vi "update file name.vi"(8 "error in":errorcluster, 11 "Picture File in":refnum<class "Picture File.lvclass">) -> (0 "error out":errorcluster, 3 "Picture File out":refnum<class "Picture File.lvclass">)   [LabVIEW 2023, in "File Classes.lvlib" / "Picture File.lvclass"]
uses:
  Picture File.lvclass
  D:/Library/LabVIEW Projects/Personal projects/Picture Organiser/PictureOrganizer/File Classes/File/File.lvclass
  Picture File.lvclass/Picture File.ctl
  File/File.lvclass/File.ctl
  File/Accessors/Read destination path.vi
  File/Accessors/Read file format.vi
  File/Read event name.vi
  File/Accessors/Read file extension.vi
  File/Accessors/Write new destination.vi
  File/File.lvclass
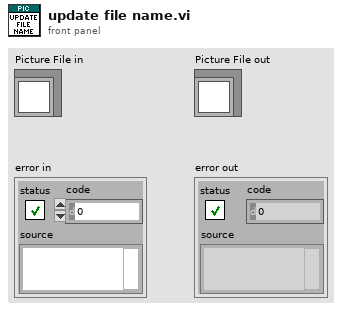
[diagram p1: front panel]
types:
  T1 = typedef "File Classes.lvlib/exif data cluster.ctl" = cluster{"Make":string, "Model":string, "Orientation":u16, "Date":timestamp, "Width":u16, "Height":u16, "Square?":bool, "File Name":string, "Extension":string, "Valid?":bool, "Path":path, "size":i64, "No Ext?":bool, "prefix?":bool, "Tag":string, "Name Type":T2, "Projection Type":string}
  T2 = typedef "File Classes.lvlib/rename type enum.ctl" = enum16{"Date & Time (Default)", "Model Sufix", "Event Sufix", "Model & Event Sufix"}
  T3 = enum16{"Date & Time (Default)", "Model Sufix", "Event Sufix", "Model & Event Sufix"}
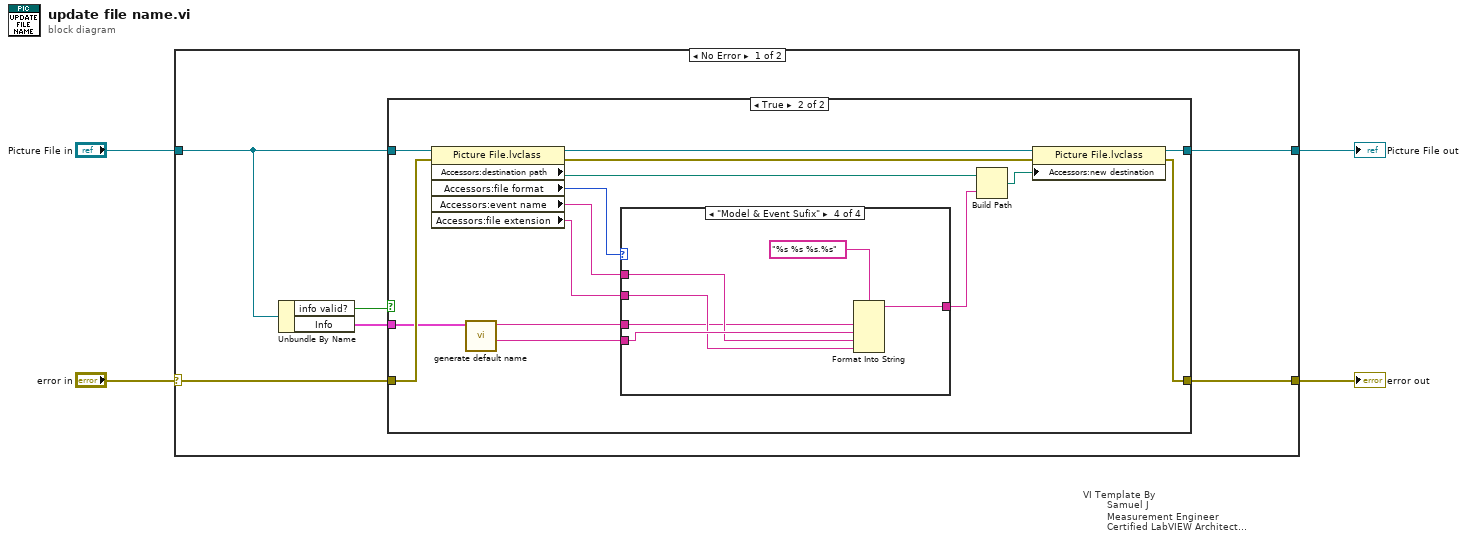
[diagram p0: block diagram]
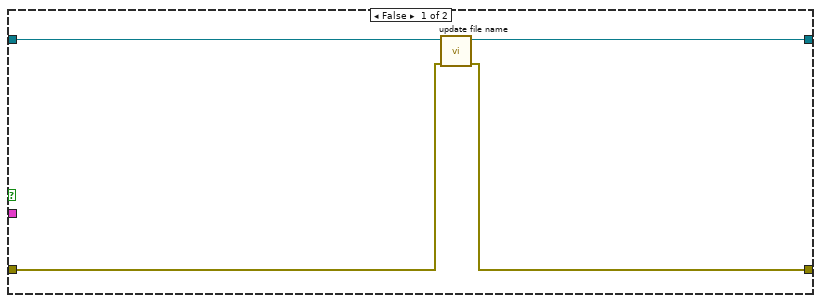
[diagram p2: hidden frame]
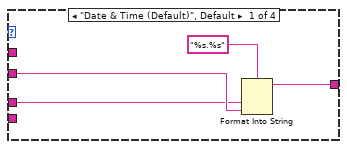
[diagram p3: hidden frame]
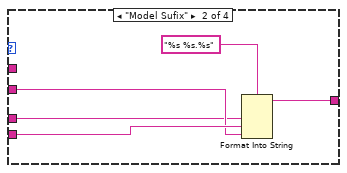
[diagram p4: hidden frame]
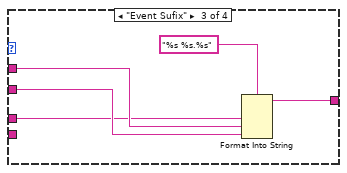
[diagram p5: hidden frame]
diagram:
  n1 = case "VI Template By\n        Samuel J\n        Measurement Engineer\n        Certified LabVIEW Architect\n        Vestas Technology R&D Chennai" shown="No Error" "error in" {
    selector: "error in" -> [w7 w51]
    tunnel: [w8 w51] -> w3
    tunnel: [w10 w50] -> w2
    tunnel: "Picture File in" -> [w9 w50]
    frame No Error {
      n2 = Unbundle By Name(w9) -> ("info valid?"=w6:bool, "Info"=w5:T1)
      n3 = case shown="True" w6 {
        tunnel: [w14 w28] -> w10
        tunnel: w9 -> [w13 w29]
        tunnel: [w11 w18] -> w8
        tunnel: w7 -> [w12 w26]
        tunnel: w5 -> [_ w17]
        frame False {
          n4 = call-parent "update file name.vi"("error in (no error)"=w12, "File in"=w13) -> ("error out"=w11:errorcluster, "File out"=w14:refnum<class "Picture File.lvclass">)  [unwired: 8 in]
        }
        frame True {
          n5 = property class="Picture File.lvclass"(reference=w29, error in=w26) -> (reference out=w27:refnum<class "Picture File.lvclass">, error out=w20:errorcluster, "Accessors:destination path"=w22:path, "Accessors:file format"=w23:T3, "Accessors:event name"=w25:string, "Accessors:file extension"=w24:string)
          n6 = call "generate default name.vi"("Info"=w17) -> ("Model"=w15:string, "default name"=w16:string)  [unwired: 9 in]
          n7 = case shown="\"Model & Event Sufix\"" w23 {
            tunnel: w25 -> [_ _ w40 w46]
            tunnel: w15 -> [_ w36 _ w47]
            tunnel: w24 -> [w31 w35 w41 w45]
            tunnel: [w32 w37 w42 w48] -> w19
            tunnel: w16 -> [w30 w34 w39 w44]
            frame "Date & Time (Default)", Default {
              n8 = Format Into String(format string="%s.%s" ("time format string (%c)"), w30, w31) -> (resulting string=w32:string)  [unwired: 2 in, 1 out]
            }
            frame "Model Sufix" {
              n9 = Format Into String(format string="%s %s.%s" ("time format string (%c)"), w34, w36, w35) -> (resulting string=w37:string)  [unwired: 2 in, 1 out]
            }
            frame "Event Sufix" {
              n10 = Format Into String(format string="%s %s.%s" ("time format string (%c)"), w39, w40, w41) -> (resulting string=w42:string)  [unwired: 2 in, 1 out]
            }
            frame "Model & Event Sufix" {
              n11 = Format Into String(format string="%s %s %s.%s" ("time format string (%c)"), w44, w47, w46, w45) -> (resulting string=w48:string)  [unwired: 2 in, 1 out]
            }
          }
          n12 = Build Path(base path=w22, name or relative path=w19) -> (appended path=w21:path)
          n13 = property class="Picture File.lvclass"(reference=w27, error in=w20, "Accessors:new destination"=w21) -> (reference out=w28:refnum<class "Picture File.lvclass">, error out=w18:errorcluster)
        }
      }
    }
    frame Error {
    }
  }
  "error out" <- w3
  "Picture File out" <- w2
